vi "CPP_Plug_in_Cross_spectraBigForVeer.vi"() -> (5 "Plug in titles":string[](array[string]), 7 "Plug in values":string[](array[string]))   [LabVIEW 2011]
uses:
  Globals/Meas_global.vi
  Globals/Plug_in_data_global.vi
panel:
  out "U1 U2 Spectra":cluster{dbl, dbl, dbl[]}[](graph)
  out "U1 U2 coherence 2":cluster{dbl, dbl, "Phase array":dbl[]}(graph)
  in  "U2":u16(ring)=1 items=["RV (Mic1)", "RV (Mic2)", "RV (Mic3)", "RV (Mic4)"]
  in  "U1":u16(ring) items=["RV (Mic1)", "RV (Mic2)", "RV (Mic3)", "RV (Mic4)"]
  in  "Display":bool=TRUE
  in  "Show Smoth":bool=TRUE
  in  "Save graphs":u16(ring) items=["Do not save plots", "Save plots"]
  out "U1 U2 phase":cluster{dbl, dbl, "Phase array":dbl[]}(graph)
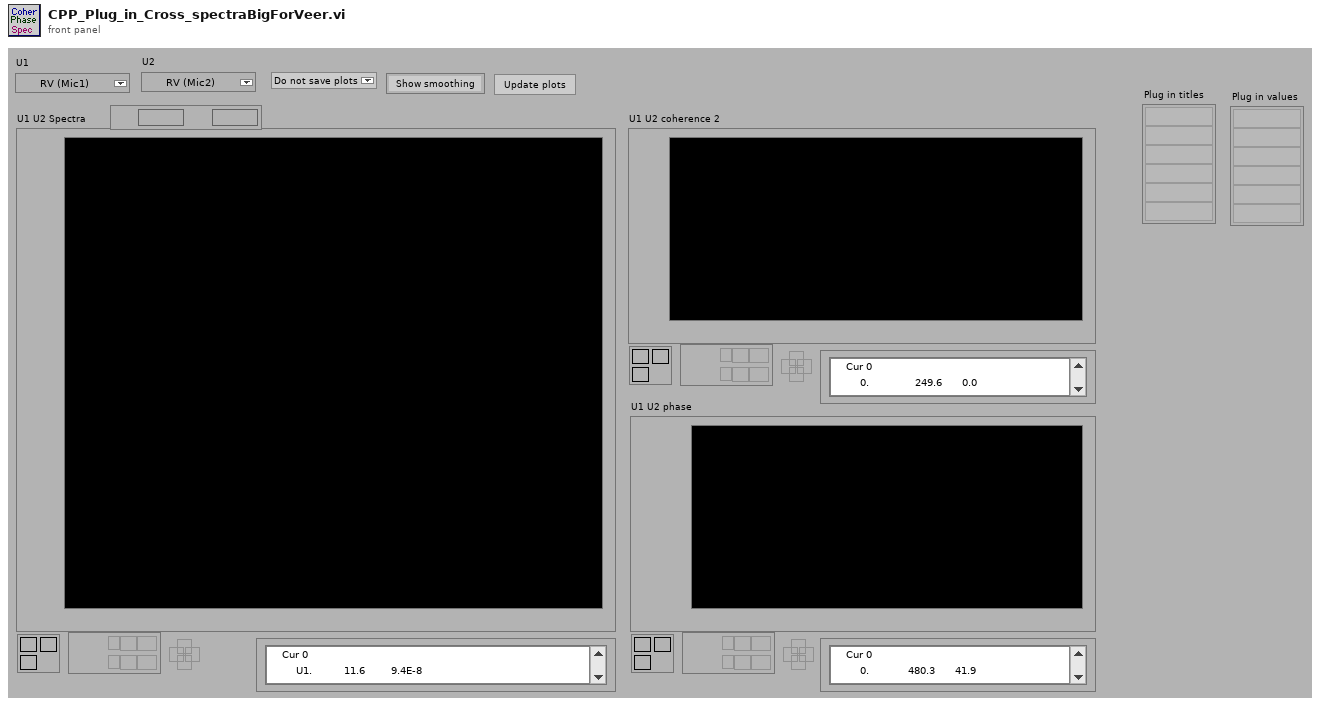
[diagram p1: front panel]
types:
  T1 = typedef "Analysis_info_cluster.ctl" = cluster{"Colour":u32, "Inst type":T2, "Inst name":string, "Symbol":string, "Code name":string, "Extra Info":string, "Inst Array":T3, "Index":i32, "Voltage Index":i32, "Extra Titles":string[], "Extra Values":string[]}
  T2 = typedef "Inst_type.ctl" = enum16{"Propeller anemometer", "Raw voltage", "Pressure Transducer", "Pitot-static tube", "Preston tube", "Hot wire", "Cross wire 1", "Cross wire 2", "Generic Linear", "Generic Polynomial", "Generic BackPoly", "Fast FID", "Thermocouple", "Cold wire", "Pulsed Wire", "LDA Vel", "LDA Tran time", "LDA Arr time"}
  T3 = typedef "Instrument_Array.ctl" = enum16{"PWA", "LDA", "Analogue"}
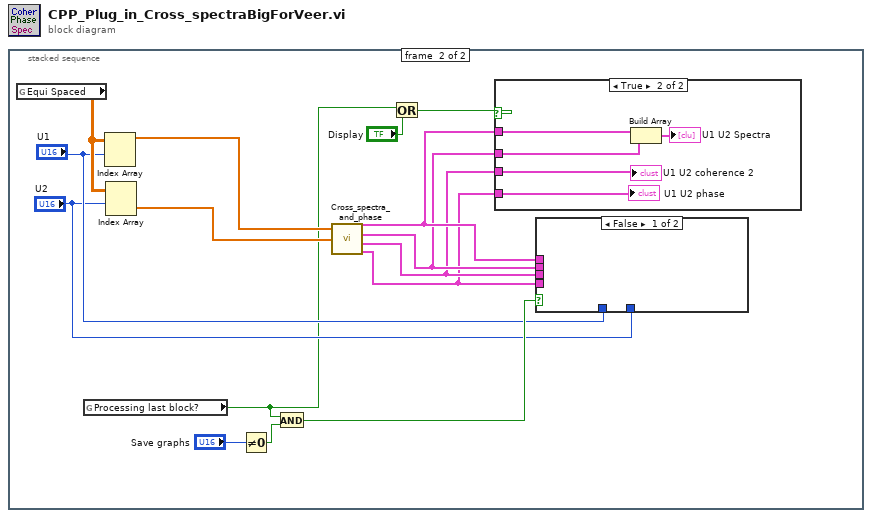
[diagram p0: block diagram]
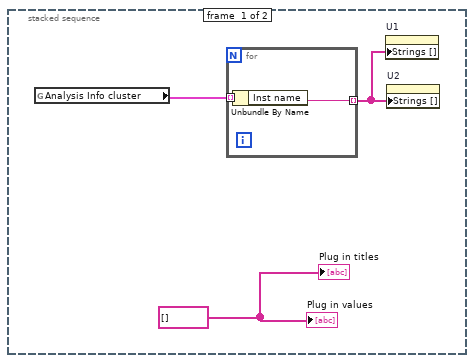
[diagram p2: hidden frame]
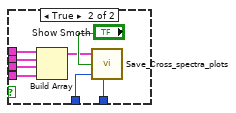
[diagram p4: hidden frame]
diagram:
  n1 = stacked-sequence {
    frame #0 {
      w1 = string[] [] ("Add in values")
      n2 = global read "Meas_global.vi" "Analysis Info cluster"() -> (w3:T1[])
      n3 = for {
        tunnel: w3 -> [w5] mode=indexing
        tunnel: [w4] -> w2 mode=indexing
        n4 = Unbundle By Name(w5) -> ("Inst name"=w4:string)
      }
      n5 = property on="U1" class="Ring (strict)"("Strings []"=w2) -> ()  [unwired: 2 in, 2 out]
      n6 = property on="U2" class="Ring (strict)"("Strings []"=w2) -> ()  [unwired: 2 in, 2 out]
      "Plug in titles" <- w1
      "Plug in values" <- w1
    }
    frame #1 {
      n7 = global read "Plug_in_data_global.vi" "Equi Spaced"() -> (w15:dbl[][])
      n8 = global read "Meas_global.vi" "Processing last block?"() -> (w6:bool)
      n9 = Index Array(array=w15, index (row)="U1") -> (element=w14:dbl[])  [unwired: 1 in]
      n10 = Index Array(array=w15, index (row)="U2") -> (element=w13:dbl[])  [unwired: 1 in]
      n11 = Not Equal To 0?(x="Save graphs") -> (x != 0?=w19:bool)
      n12 = And(x=w6, y=w19) -> (x .and. y?=w18:bool)
      n13 = call "Cross_spectra_and_phase.vi"("U1"=w14, "U2"=w13) -> ("U1 spectra"=w10:cluster{dbl, dbl, dbl[]}, "U2 spectra"=w9:cluster{dbl, dbl, dbl[]}, "U1 U2 coherence"=w8:cluster{dbl, dbl, "Coherence array":dbl[]}, "U1 U2 phase"=w7:cluster{dbl, dbl, "Phase array":dbl[]})  [unwired: 3 out]
      n14 = Or(x=w6, y="Display") -> (x .or. y?=w17:bool)
      n15 = case shown="True" w17 {
        tunnel: w10 -> [_ w23]
        tunnel: w9 -> [_ w22]
        tunnel: w8 -> [_ w24]
        tunnel: w7 -> [_ w25]
        frame False {
        }
        frame True {
          n16 = Build Array(w23, w22) -> (→"U1 U2 Spectra":cluster{dbl, dbl, dbl[]}[])
          "U1 U2 phase" <- w25
          "U1 U2 coherence 2" <- w24
        }
      }
      n17 = case shown="False" w18 {
        tunnel: "U1" -> [_ w32]
        tunnel: "U2" -> [_ w31]
        tunnel: w10 -> [_ w29]
        tunnel: w9 -> [_ w28]
        tunnel: w8 -> [_ w27]
        tunnel: w7 -> [_ w26]
        frame False {
        }
        frame True {
          n18 = Build Array(w29, w28, w27, w26) -> (w30:cluster{dbl, dbl, "Phase array":dbl[]}[])
          n19 = call "Save_Cross_spectra_plots.vi"("Plots to save"=w30, "Show Smooth"="Show Smoth", "U1"=w32, "U2"=w31) -> ()  [unwired: 1 in, 2 out]
        }
      }
    }
  }
